vi "Flock_Master_IncrementRev.vi"(8 "error in (no error)":errorcluster) -> (0 "error out":errorcluster)   [LabVIEW 2013, in "Flock_Master_BuildRevision.lvlib"]
uses:
  Flock_Master_BuildRevision.lvlib
panel:
  in  "Cancel Button":bool
  out "BranchNum":i32
  in  "BranchNum":i32
  in  "Build":bool
  in  "BuildPhase":string
  in  "BuildNum":i32
  in  "MinorRev":i32
  in  "MajorRev":i32
  out "BuildPhase":string
  out "BuildNum":i32
  out "MinorRev":i32
  out "MajorRev":i32
  in  "configuration file path":path=path "C:/Users/Mark Black/Perforce/penguin_1666/mblack_PerforceWin/user/mblack/Flock/trunk/Shared Resources/static/FlockRev.ini"
  # "Previous Build"
  # "New Build"
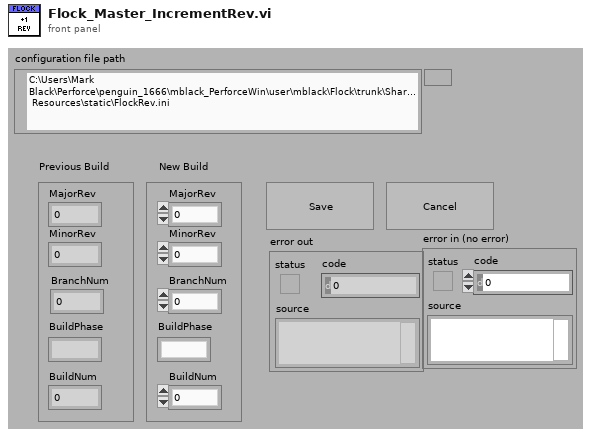
[diagram p1: front panel]
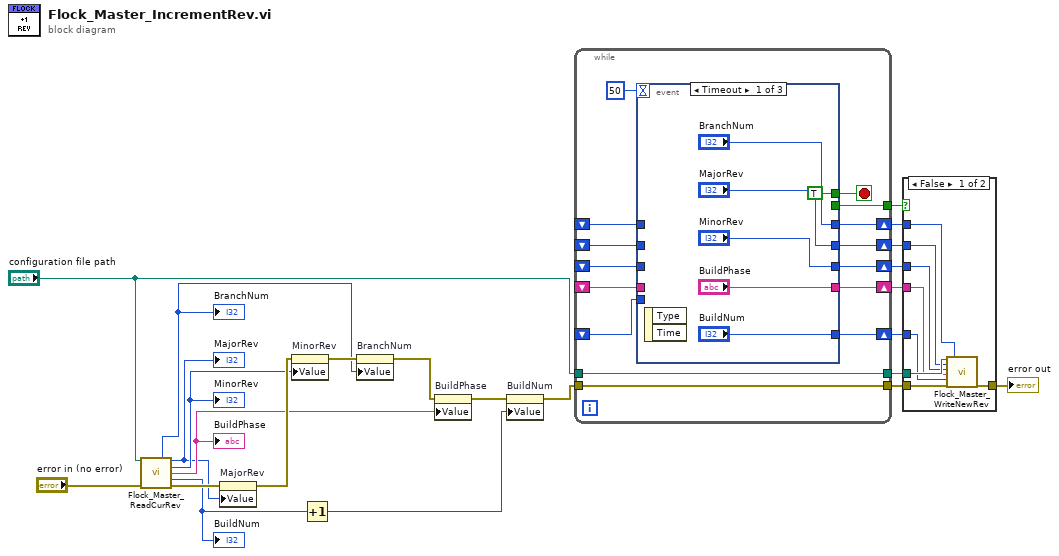
[diagram p0: block diagram]
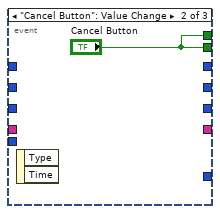
[diagram p3: hidden frame]
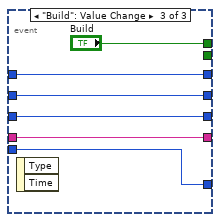
[diagram p4: hidden frame]
diagram:
  n1 = call "Flock_Master_ReadCurRev.vi"("configuration file path"="configuration file path", "error in (no error)"="error in (no error)") -> ("BranchNum"=w5:i32, "MajorRev"=w8:i32, "MinorRev"=w9:i32, "BuildPhase"=w10:string, "BuildNum"=w11:i32, "error out"=w13:errorcluster)  [unwired: 8 in]
  "MajorRev" <- w8
  "MinorRev" <- w9
  "BuildNum" <- w11
  "BuildPhase" <- w10
  "BranchNum" <- w5
  n2 = property on="MajorRev" class="DigNum (strict)"(error in=w13, "Value"=w8) -> (error out=w23:errorcluster)  [unwired: 1 in, 1 out]
  n3 = property on="MinorRev" class="DigNum (strict)"(error in=w23, "Value"=w9) -> (error out=w6:errorcluster)  [unwired: 1 in, 1 out]
  n4 = Increment(x=w11) -> (x+1=w20:i32)
  n5 = property on="BranchNum" class="DigNum (strict)"(error in=w6, "Value"=w5) -> (error out=w4:errorcluster)  [unwired: 1 in, 1 out]
  n6 = property on="BuildPhase" class="Str"(error in=w4, "Value"=w10) -> (error out=w22:errorcluster)  [unwired: 1 in, 1 out]
  n7 = property on="BuildNum" class="DigNum (strict)"(error in=w22, "Value"=w20) -> (error out=w21:errorcluster)  [unwired: 1 in, 1 out]
  n8 = while {
    tunnel: w21 -> [w32]
    tunnel: "configuration file path" -> [w38]
    tunnel: [w38] -> w19
    tunnel: [w32] -> w14
    shift-right: [w36] -> w18
    shift-left: _ -> [w28]
    shift-right: [w35] -> w17
    shift-left: _ -> [w29]
    shift-right: [w34] -> w16
    shift-left: _ -> [w30]
    shift-right: [w33] -> w15
    shift-left: _ -> [w31]
    shift-right: [w27] -> w7
    shift-left: _ -> [w26]
    tunnel: [w24] -> w3
    stop <- w25 stop-if-true
    n9 = event shown="[0] Timeout" {
      selector: _ -> [_ _ _]
      dyn-events: _ -> [_ _ _]
      timeout: 50 ("Numeric") -> [_ _ _]
      tunnel: [TRUE ("Build") "Cancel Button" "Build"] -> w25
      tunnel: ["MajorRev" _ w47] -> w36
      tunnel: ["MinorRev" _ w48] -> w35
      tunnel: ["BuildPhase" _ w49] -> w34
      tunnel: ["BuildNum" _ w50] -> w33
      tunnel: w31 -> [_ _ w50]
      tunnel: w30 -> [_ _ w49]
      tunnel: w29 -> [_ _ w48]
      tunnel: w28 -> [_ _ w47]
      tunnel: ["BranchNum" _ w46] -> w27
      tunnel: w26 -> [_ _ w46]
      tunnel: [_ "Cancel Button" _] -> w24
      event Timeout {
        n10 = event-data() -> ()  [unwired: 1 in, 2 out]
      }
      event "Cancel Button": Value Change {
        n11 = event-data() -> ()  [unwired: 1 in, 2 out]
      }
      event "Build": Value Change {
        n12 = event-data() -> ()  [unwired: 1 in, 2 out]
      }
    }
  }
  n13 = case shown="False" w3 {
    tunnel: w19 -> [w59 _]
    tunnel: w18 -> [w58 _]
    tunnel: w17 -> [w57 _]
    tunnel: w16 -> [w56 _]
    tunnel: w15 -> [w55 _]
    tunnel: w14 -> [w54 w60]
    tunnel: w7 -> [w53 _]
    tunnel: [w52 w60] -> w2
    frame False {
      n14 = call "Flock_Master_WriteNewRev.vi"("configuration file path"=w59, "MajorRev"=w58, "MinorRev"=w57, "BuildPhase"=w56, "BuildNum"=w55, "error in (no error)"=w54, "BranchNum"=w53) -> ("error out"=w52:errorcluster)  [unwired: 12 in]
    }
    frame True {
    }
  }
  "error out" <- w2
